vi "GetQ_single enum.vi"(8 "error in (no error)":errorcluster, 10 "Enum":variant) -> (0 "error out":errorcluster, 1 "found":bool, 2 "Queue":refnum<queue>)   [LabVIEW 2020, in "QDict.lvlib"]
doc: "Developed by Kevin Thompson\nkevin@thompsonengineering.net\n\nCopyright 2021\nThompson Engineering, LLC"
uses:
  QDict.lvlib
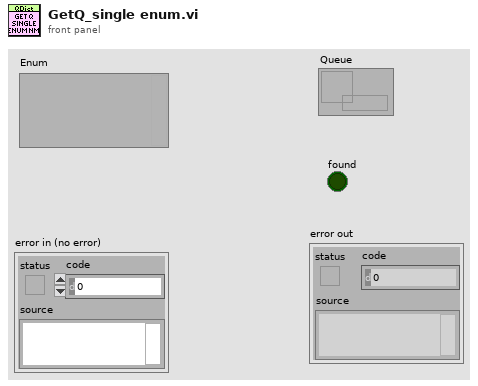
[diagram p1: front panel]
types:
  T1 = typedef "Type Descriptor Enumeration__ogtk.ctl" = enum8{"<Null>", "I8", "I16", "I32", "I64", "U8", "U16", "U32", "U64", "SGL", "DBL", "EXT", "CSG", "CDB", "CXT", "0x0F", "0x10", "0x11", "0x12", "0x13", "0x14", "Enum U8", "Enum U16", "Enum U32", "Enum U64", "SGL PQ", "DBL PQ", "EXT PQ", "CSG PQ", "CDB PQ", "CXT PQ", "0x1F", "0x20", "Boolean", "0x22", "0x23", "0x24", "0x25", "0x26", "0x27", "0x28", "0x29", "0x2A", "0x2B", "0x2C", "0x2D", "0x2E", "0x2F", "String", "0x31", "Path", "Pict", "0x34", "0x35", "0x36", "DAQ", "0x38", "0x39", "0x3A", "0x3B", "0x3C", "0x3D", "0x3E", "0x3F", "Array", "0x41", "0x42", "0x43", "0x44", "0x45", "0x46", "0x47", "0x48", "0x49", "0x4A", "0x4B", "0x4C", "0x4D", "0x4E", "0x4F", "Cluster", "0x51", "0x52", "Variant", "Waveform", "0x55", "0x56", "0x57", "0x58", "0x59", "0x5A", "0x5B", "0x5C", "0x5D", "0x5E", "0x5F", "0x60", "0x61", "0x62", "0x63", "0x64", "0x65", "0x66", "0x67", "0x68", "0x69", "0x6A", "0x6B", "0x6C", "0x6D", "0x6E", "0x6F", "Refnum"}
  T2 = typedef "TD Dynamic CVT DVR--ref.ctl" = refnum<data-value>
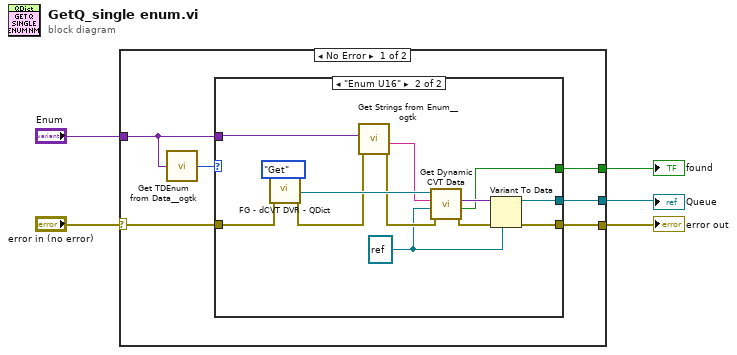
[diagram p0: block diagram]
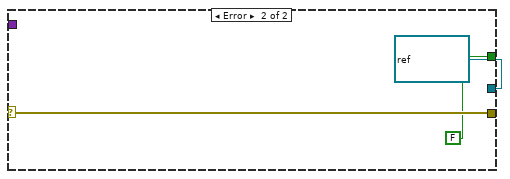
[diagram p3: hidden frame]
diagram:
  n1 = case shown="No Error" "error in (no error)" {
    selector: "error in (no error)" -> [w11 w28]
    tunnel: [w10 w28] -> w5
    tunnel: "Enum" -> [w8 _]
    tunnel: [w7 refnum<queue> refnum ("queue out")] -> w1
    tunnel: [w6 FALSE ("found")] -> w2
    frame No Error {
      n2 = call <userlib>:"Get TDEnum from Data__ogtk.vi"("Data"=w8) -> ("Type Descriptor Enumeration"=w9:T1)  [unwired: 4 in]
      n3 = case shown="\"Enum U16\"" w9 {
        tunnel: w11 -> [w12 w20]
        tunnel: [w12 w25] -> w10
        tunnel: w8 -> [_ w21]
        tunnel: [_ w15] -> w7
        tunnel: [_ w14] -> w6
        frame "<Null>", Default {
        }
        frame "Enum U16" {
          w13 = refnum<queue> refnum ("queue out")
          n4 = call "FG - dCVT DVR - QDict.vi"("error in (no error)"=w20, "Action (Get)"=enum16{"Init", "Get", "Set"}."Get") -> ("dCVT QMH out"=w23:T2, "error out"=w22:errorcluster)  [unwired: 7 in]
          n5 = call <userlib>:"Get Strings from Enum__ogtk.vi"("error in (no error)"=w22, "Enum"=w21) -> ("error out"=w16:errorcluster, "String Value"=w17:string)  [unwired: 6 in, 2 out]
          n6 = call <vilib>:"Get Dynamic CVT Data.vi"("error in (no error)"=w16, "default value (empty variant)"=w13, "DataName"=w17, "dCVT DVR"=w23) -> ("error out"=w19:errorcluster, "found"=w14:bool, "value"=w18:variant)  [unwired: 4 in, 1 out]
          n7 = Variant To Data(error in=w19, type=w13, Variant=w18) -> (data=w15:refnum<queue>, error out=w25:errorcluster)
        }
      }
    }
    frame Error {
    }
  }
  "error out" <- w5
  "Queue" <- w1
  "found" <- w2
